vi "MDriveCommand.vi"(4 "Channel Name":string, 6 "Port Name":string, 8 "Numeric Value":dbl format="%.2f", 9 "MDriveCommand":T2="DePowerMotor", 10 "Address":i8) -> (0 "String Reply":string, 1 "Error Description":string, 2 "Numeric Reply":dbl, 3 "OK":bool)   [LabVIEW 2020]
uses:
  MDriveDriveCommand.ctl
  CommandDescriptor.ctl
  ~subVIs/CommandPhases.ctl
  ~subVIs/GenericDriveCommand.ctl
panel:
  out "CommandDescriptorOutput":T1
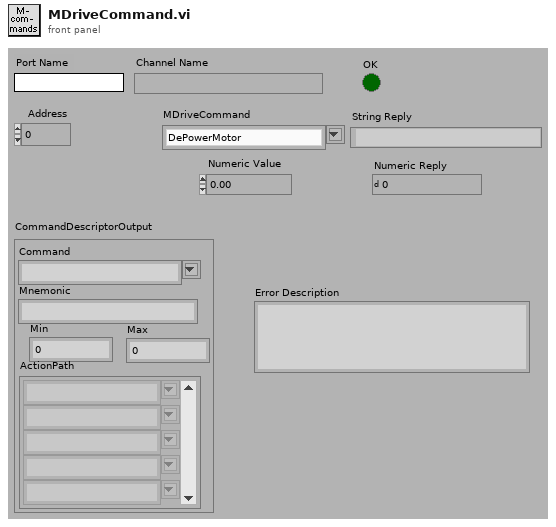
[diagram p1: front panel]
types:
  T1 = typedef "CommandDescriptor.ctl" = cluster{"Command":T2, "Mnemonic":string, "Min":dbl, "Max":dbl, "ActionPath":T3[]}
  T2 = typedef "MDriveDriveCommand.ctl" = string
  T3 = typedef "CommandPhases.ctl" = string
  T4 = typedef "GenericDriveCommand.ctl" = string
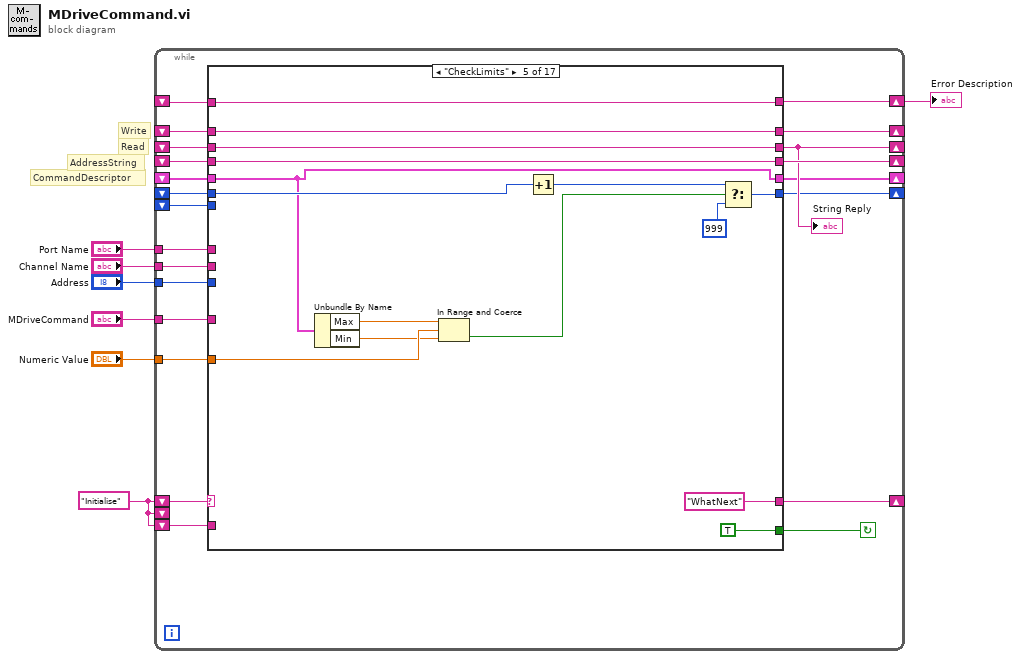
[diagram p0: block diagram]
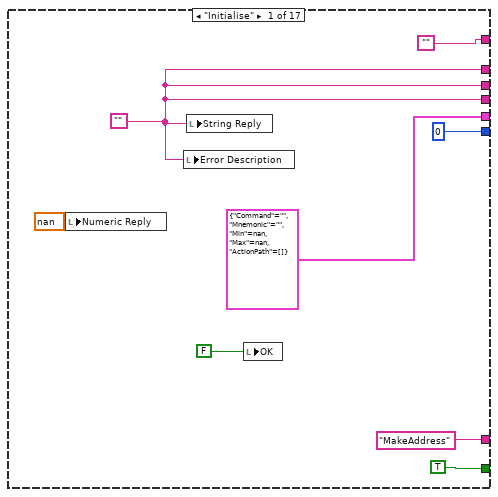
[diagram p2: hidden frame]
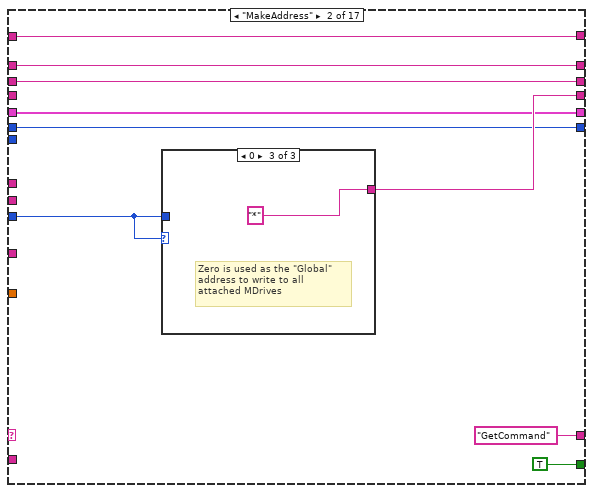
[diagram p3: hidden frame]
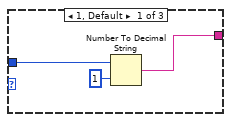
[diagram p4: hidden frame]
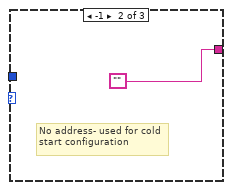
[diagram p5: hidden frame]
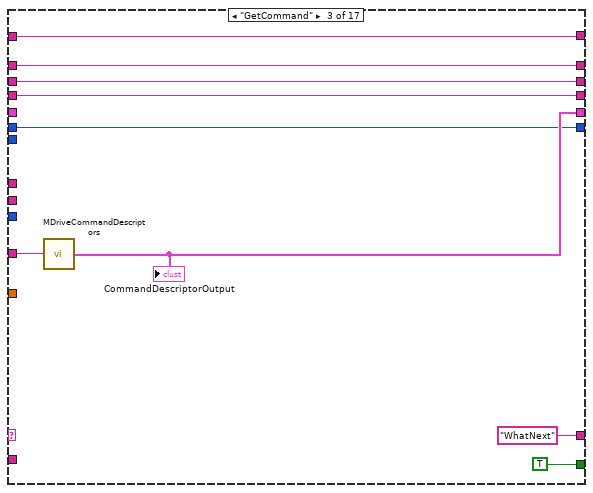
[diagram p6: hidden frame]
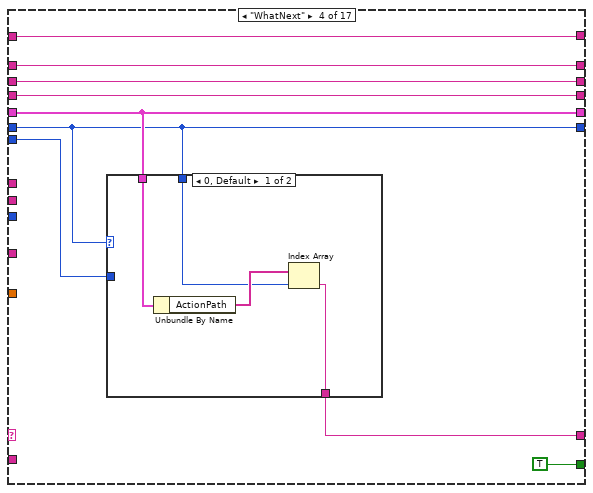
[diagram p7: hidden frame]
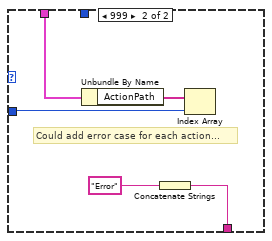
[diagram p8: hidden frame]
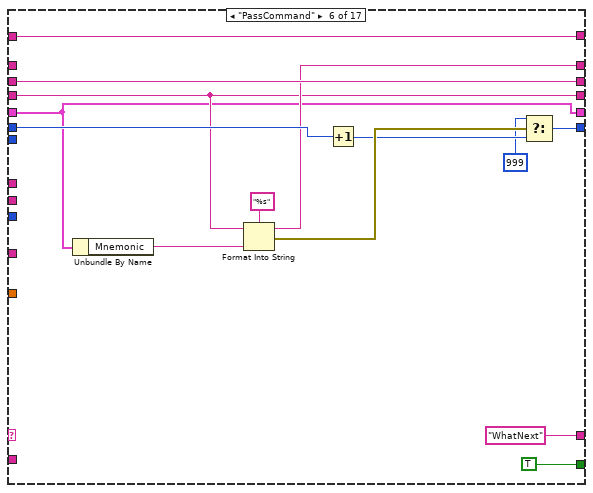
[diagram p9: hidden frame]
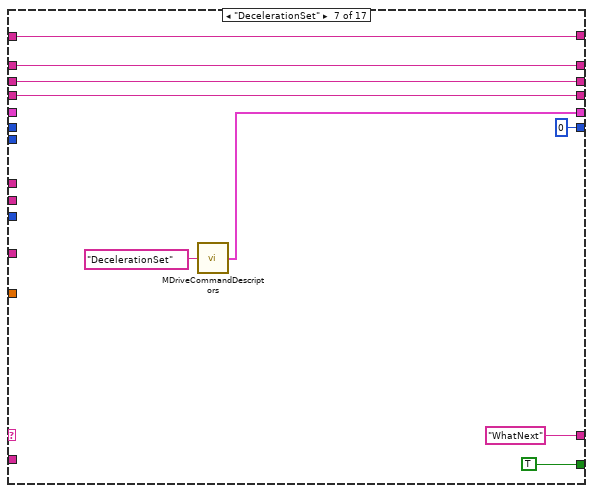
[diagram p10: hidden frame]
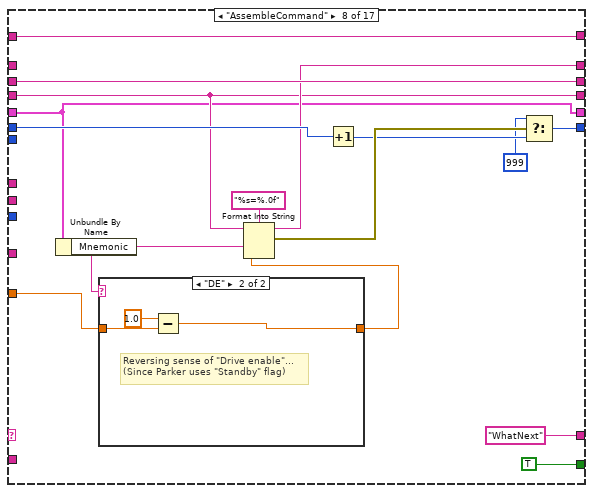
[diagram p11: hidden frame]
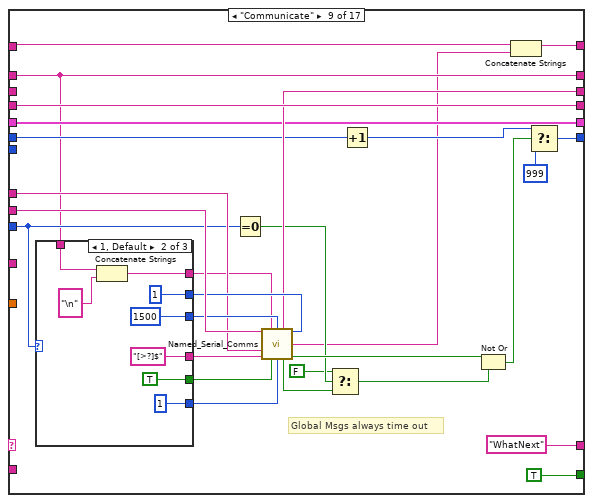
[diagram p13: hidden frame]
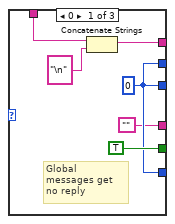
[diagram p14: hidden frame]
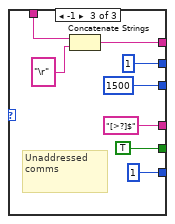
[diagram p15: hidden frame]
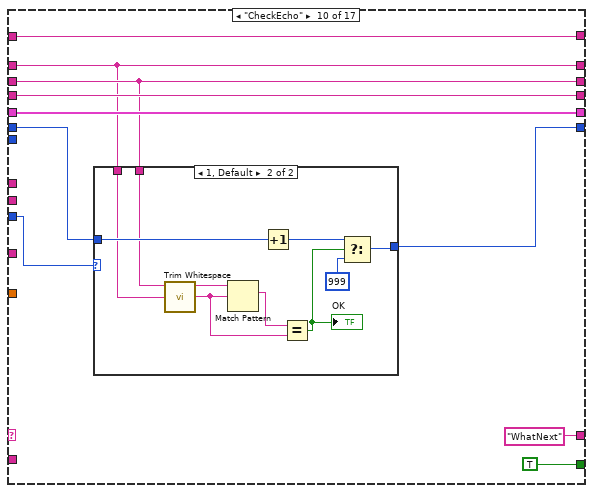
[diagram p16: hidden frame]
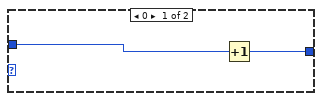
[diagram p17: hidden frame]
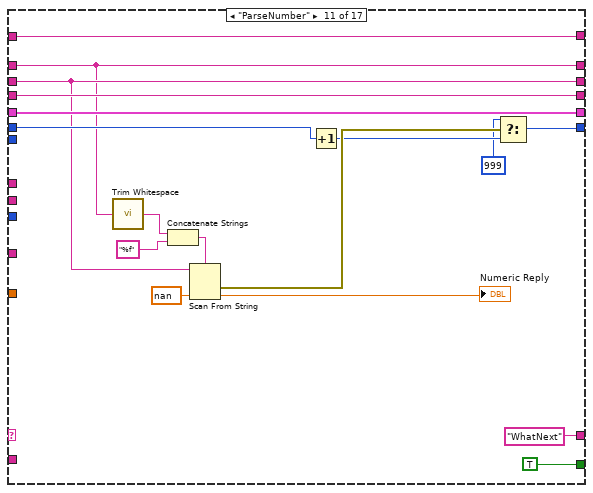
[diagram p18: hidden frame]
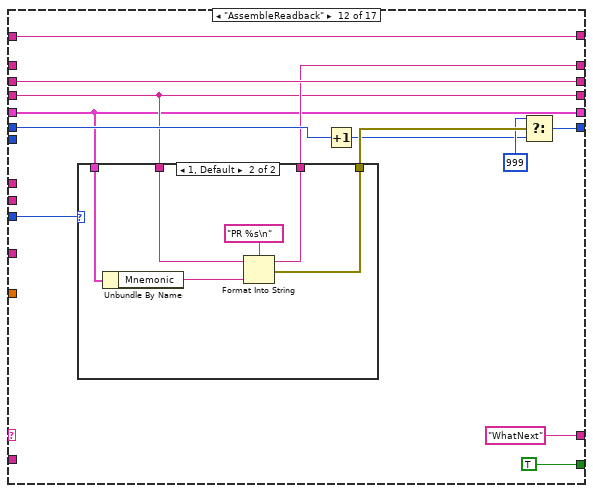
[diagram p19: hidden frame]
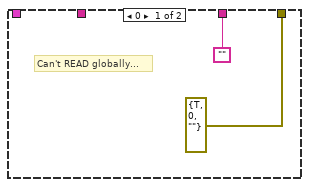
[diagram p20: hidden frame]
diagram:
  w2 = "Initialise"
  # "CommandDescriptor"
  # "AddressString"
  # "Read"
  # "Write"
  n1 = while {
    shift-right: [w18] -> _
    shift-left: w2 -> [w12]
    tunnel: "Address" -> [w29]
    tunnel: "MDriveCommand" -> [w28]
    tunnel: "Numeric Value" -> [w27]
    shift-right: [w26] -> _
    shift-left: _ -> [w25]
    tunnel: "Port Name" -> [w24]
    tunnel: "Channel Name" -> [w23]
    shift-right: [w17] -> _
    shift-left: _ -> [w22]
    shift-right: [w20] -> _
    shift-left: _ -> [w19]
    shift-right: [w16] -> _
    shift-left: _ -> [w15]
    shift-right: [w13] -> _
    shift-left: _ -> [w14]
    shift-left: _ -> [w11]
    shift-left: w2 -> [_]
    shift-left: w2 -> [w10]
    shift-right: [w8] -> w1
    shift-left: _ -> [w9]
    stop <- w21 continue-if-true
    n2 = case shown="\"CheckLimits\"" w12 {
      selector: w12 -> [_ _ _ _ _ _ _ _ _ _ _ _ _ _ _ _ w324]
      tunnel: ["MakeAddress" "GetCommand" "WhatNext" w65 "WhatNext" "WhatNext" "WhatNext" "WhatNext" "WhatNext" "WhatNext" "WhatNext" "WhatNext" w250 "Error" "Initialise" "Initialise" w324] -> w18
      tunnel: w29 -> [_ w39 _ _ _ _ _ _ w142 w188 _ w229 _ _ _ _ _]
      tunnel: w28 -> [_ _ w57 _ _ _ _ _ _ _ _ _ _ _ _ _ _]
      tunnel: w27 -> [_ _ _ _ w91 _ _ w119 _ _ _ _ _ _ _ w311 _]
      tunnel: [w32 w44 w59 w68 w89 w102 w110 w127 w141 w189 w211 w232 w256 w274 w303 w316 w322] -> w26
      tunnel: w25 -> [_ w44 w59 w68 w89 _ w110 _ w141 w189 w211 _ w256 w274 w296 _ _]
      tunnel: w24 -> [_ _ _ _ _ _ _ _ w158 _ _ _ _ _ w297 _ _]
      tunnel: w23 -> [_ _ _ _ _ _ _ _ w164 _ _ _ _ w269 w298 _ _]
      tunnel: [w32 w43 w58 w67 w93 w107 w116 w132 w155 w190 w218 w237 w254 w279 w303 w316 w322] -> w17
      tunnel: w22 -> [_ w43 w58 w67 w93 w107 w116 w132 _ w190 w218 w237 w254 w279 w295 _ _]
      tunnel: [TRUE TRUE ("Continue") TRUE ("Continue") TRUE ("Continue") TRUE TRUE TRUE TRUE TRUE TRUE TRUE TRUE w251 TRUE FALSE ("Continue") FALSE ("Continue") FALSE] -> w21
      tunnel: [w32 w46 w56 w66 w92 w101 w113 w126 w156 w195 w223 w230 w255 w284 w303 w316 w322] -> w20
      tunnel: w19 -> [_ _ w56 w66 w92 w101 w113 w126 w156 w195 w223 w230 w255 w284 _ w309 _]
      tunnel: [T1 {"Command"="", "Mnemonic"="", "Min"=nan, "Max"=nan, "ActionPath"=[]} ("CommandDescriptorOutput") w41 w54 w64 w80 w98 w112 w124 w154 w191 w219 w228 w248 w280 w302 w314 w321] -> w16
      tunnel: w15 -> [_ w41 _ w64 w80 w98 _ w124 w154 w191 w219 w228 w247 w280 w302 w314 w321]
      tunnel: w14 -> [_ w40 w53 w63 w84 w103 _ w128 w149 w192 w220 w233 _ w281 w301 w315 w320]
      tunnel: [0 w40 w53 w63 w85 w104 0 ("f") w129 w151 w193 w221 w234 0 ("f") w282 w301 w315 w320] -> w13
      tunnel: w11 -> [_ _ _ w62 _ _ _ _ _ _ _ _ _ _ _ _ _]
      tunnel: w10 -> [_ _ _ _ _ _ _ _ _ _ _ _ _ _ w293 _ _]
      tunnel: w9 -> [_ w38 w52 w61 w79 w94 w108 w117 w139 w187 w208 w225 w246 w266 w286 w308 w319]
      tunnel: ["" w38 w52 w61 w79 w94 w108 w117 w138 w187 w208 w225 w246 w264 w286 w306 w319] -> w8
      frame "Initialise" {
        w32 = ""
        n3 = local write "Numeric Reply"(nan ("Numeric Reply")) -> ()
        n4 = local write "Error Description"(w32) -> ()
        n5 = local write "String Reply"(w32) -> ()
        n6 = local write "OK"(FALSE ("GoodEcho")) -> ()
      }
      frame "MakeAddress" {
        n7 = case shown="0" w39 {
          tunnel: w39 -> [w48 _ _]
          tunnel: [w47 "" "*"] -> w46
          frame 1, Default {
            n8 = Number To Decimal String(number=w48, width (-)=i16 1) -> (decimal integer string=w47:string)
          }
          frame -1 {
            # "No address- used for cold start configuration"
          }
          frame 0 {
            # "Zero is used as the \"Global\" address to write to all attached MDrives"
          }
        }
      }
      frame "GetCommand" {
        n9 = call "MDriveCommandDescriptors.vi"("MDriveCommand"=w57) -> ("CommandDescriptorOutput"=w54:T1)  [unwired: 4 out]
        "CommandDescriptorOutput" <- w54
      }
      frame "WhatNext" {
        n10 = case shown="0, Default" w63 {
          tunnel: [w72 w75] -> w65
          tunnel: w64 -> [w71 w76]
          tunnel: w63 -> [w70 _]
          tunnel: w62 -> [_ w77]
          frame 0, Default {
            n11 = Unbundle By Name(w71) -> ("ActionPath"=w73:T3[])
            n12 = Index Array(array=w73, index=w70) -> (element=w72:T3)
          }
          frame 999 {
            # "Could add error case for each action..."
            n13 = Unbundle By Name(w76) -> ("ActionPath"=w78:T3[])
            n14 = Concatenate Strings("Error") -> (w75:string)
            n15 = Index Array(array=w78, index=w77) -> ()  [unwired: 1 out]
          }
        }
      }
      frame "CheckLimits" {
        n16 = Unbundle By Name(w80) -> ("Max"=w88:dbl, "Min"=w87:dbl)
        n17 = In Range and Coerce(upper limit=w88, x=w91, lower limit=w87) -> (In Range?=w82:bool)  [unwired: 1 out]
        n18 = Increment(x=w84) -> (x+1=w83:i32)
        n19 = Select(t=w83, s=w82, f=999) -> (s? t:f=w85:i32)
      }
      frame "PassCommand" {
        n20 = Unbundle By Name(w98) -> ("Mnemonic"=w100:string)
        n21 = Format Into String(format string="%s", initial string=w101, w100) -> (resulting string=w102:string, error out=w97:errorcluster)  [unwired: 1 in]
        n22 = Increment(x=w103) -> (x+1=w96:i32)
        n23 = Select(t=999 ("f"), s=w97, f=w96) -> (s? t:f=w104:i32)
      }
      frame "DecelerationSet" {
        n24 = call "MDriveCommandDescriptors.vi"("MDriveCommand"=T4 "DecelerationSet" ("GenericDriveCommand")) -> ("CommandDescriptorOutput"=w112:T1)  [unwired: 4 out]
      }
      frame "AssembleCommand" {
        n25 = Unbundle By Name(w124) -> ("Mnemonic"=w120:string)
        n26 = case shown="\"DE\"" w120 {
          tunnel: w119 -> [w133 w136]
          tunnel: [w133 w134] -> w118
          frame "False", Default {
          }
          frame "DE" {
            # "Reversing sense of \"Drive enable\"...\n(Since Parker uses \"Standby\" flag)"
            n27 = Subtract(x=1.0, y=w136) -> (x-y=w134:dbl)
          }
        }
        n28 = Format Into String(format string="%s=%.0f", initial string=w126, w120, w118) -> (resulting string=w127:string, error out=w123:errorcluster)  [unwired: 1 in]
        n29 = Increment(x=w128) -> (x+1=w122:i32)
        n30 = Select(t=999 ("f"), s=w123, f=w122) -> (s? t:f=w129:i32)
      }
      frame "Communicate" {
        # "Global Msgs always time out"
        n31 = case shown="1, Default" w142 {
          tunnel: ["" "[>?]$" "[>?]$"] -> w163
          tunnel: [w169 1 ("Terminate Count") 1 ("Terminate Count")] -> w162
          tunnel: [w169 u32 1500 ("Timeout/ms") u32 1500 ("Timeout/ms")] -> w161
          tunnel: [TRUE ("Log Errors?") TRUE ("Log Errors?") TRUE ("Log Errors?")] -> w160
          tunnel: [w169 1 ("!Error retries") 1 ("!Error retries")] -> w159
          tunnel: w141 -> [w165 w173 w181]
          tunnel: [w166 w172 w180] -> w140
          frame 0 {
            w169 = 0 ("!Error retries")
            # "Global messages get no reply"
            n32 = Concatenate Strings(w165, "\n" ("string")) -> (w166:string)
          }
          frame 1, Default {
            n33 = Concatenate Strings(w173, "\n" ("string")) -> (w172:string)
          }
          frame -1 {
            # "Unaddressed comms"
            n34 = Concatenate Strings(w181, "\r" ("string")) -> (w180:string)
          }
        }
        n35 = Equal To 0?(x=w142) -> (x = 0?=w145:bool)
        n36 = call "Named_Serial_Comms.vi"("Channel Name"=w164, "Write"=w140, "Timeout/ms"=w161, "!Error retries"=w159, "Port Name"=w158, "Term Grep"=w163, "Log Errors?"=w160, "Terminate Count"=w162) -> ("Read"=w155:string, "Error Description"=w137:string, "Timed out"=w144:bool, "Serial Error"=w152:bool)  [unwired: 1 in, 3 out]
        n37 = Select(t=FALSE, s=w145, f=w144) -> (s? t:f=w146:bool)
        n38 = Increment(x=w149) -> (x+1=w148:i32)
        n39 = Not Or(1:w146, 2:w152) -> (0:w150:bool)
        n40 = Concatenate Strings(w139, w137) -> (w138:string)
        n41 = Select(t=w148, s=w150, f=999) -> (s? t:f=w151:i32)
      }
      frame "CheckEcho" {
        n42 = case shown="1, Default" w188 {
          tunnel: [w197 w206] -> w193
          tunnel: w192 -> [w198 w203]
          tunnel: w190 -> [_ w201]
          tunnel: w189 -> [_ w200]
          frame 0 {
            n43 = Increment(x=w198) -> (x+1=w197:i32)
          }
          frame 1, Default {
            n44 = call <vilib>:"Trim Whitespace.vi"("string"=w200) -> ("trimmed string"=w199:string)  [unwired: 1 in]
            n45 = Match Pattern(string=w201, regular expression=w199) -> (match substring=w202:string)  [unwired: 4 out]
            n46 = Increment(x=w203) -> (x+1=w204:i32)
            n47 = Equal?(x=w202, y=w199) -> (x = y?=w205:bool)
            "OK" <- w205
            n48 = Select(t=w204, s=w205, f=999) -> (s? t:f=w206:i32)
          }
        }
      }
      frame "ParseNumber" {
        n49 = call <vilib>:"Trim Whitespace.vi"("string"=w211) -> ("trimmed string"=w209:string)  [unwired: 1 in]
        n50 = Concatenate Strings(w209, "%f" ("format string")) -> (w212:string)
        n51 = Scan From String(format string=w212, input string=w218, default 1=nan ("default value 1")) -> (error out=w216:errorcluster, output 1=→"Numeric Reply":dbl)  [unwired: 2 in, 2 out]
        n52 = Increment(x=w220) -> (x+1=w215:i32)
        n53 = Select(t=999, s=w216, f=w215) -> (s? t:f=w221:i32)
      }
      frame "AssembleReadback" {
        n54 = case shown="1, Default" w229 {
          tunnel: w228 -> [_ w245]
          tunnel: ["" w244] -> w232
          tunnel: [errorcluster {"status"=TRUE, "code"=0, "source"=""} ("error IO") w243] -> w231
          tunnel: w230 -> [_ w242]
          frame 0 {
            # "Can't READ globally..."
          }
          frame 1, Default {
            n55 = Unbundle By Name(w245) -> ("Mnemonic"=w241:string)
            n56 = Format Into String(format string="PR %s\n", initial string=w242, w241) -> (resulting string=w244:string, error out=w243:errorcluster)  [unwired: 1 in]
          }
        }
        n57 = Increment(x=w233) -> (x+1=w226:i32)
        n58 = Select(t=999 ("f"), s=w231, f=w226) -> (s? t:f=w234:i32)
      }
      frame "Done" {
        n59 = Match Pattern(string=w254, regular expression="?") -> (offset past match=w249:i32)  [unwired: 4 out]
        n60 = case shown="-1" w249 {
          tunnel: [TRUE ("Continue") FALSE ("Continue")] -> w251
          tunnel: ["WhatNext" "Initialise"] -> w250
          tunnel: [w259 w261] -> w248
          tunnel: w247 -> [_ w261]
          frame 0, Default {
            n61 = call "MDriveCommandDescriptors.vi"("MDriveCommand"=T4 "GetError" ("GenericDriveCommand")) -> ("CommandDescriptorOutput"=w259:T1)  [unwired: 4 out]
          }
          frame -1 {
          }
        }
      }
      frame "ParseError" {
        n62 = call <vilib>:"Trim Whitespace.vi"("string"=w274) -> ("trimmed string"=w272:string)  [unwired: 1 in]
        n63 = Concatenate Strings(w272, "%s" ("format string")) -> (w275:string)
        n64 = Scan From String(format string=w275, input string=w279, default 1="") -> (error out=w278:errorcluster, output 1=w270:string)  [unwired: 2 in, 2 out]
        n65 = call "MDriveErrorCodes.vi"("Error Code"=w270) -> ("Error Description"=w268:string)  [unwired: 4 out]
        n66 = Increment(x=w281) -> (x+1=w277:i32)
        n67 = Format Into String(format string="The %s has %s", w269, w268) -> (resulting string=w265:string)  [unwired: 2 in, 1 out]
        n68 = Concatenate Strings(w266, w265) -> (w264:string)
        n69 = Select(t=999, s=w278, f=w277) -> (s? t:f=w282:i32)
      }
      frame "Error" {
        w290 = "Error in MDriveCommand.vi: " ("string")
        w303 = ""
        n70 = local read "Error Description"() -> (w289:string)
        n71 = call "Serial_log_build.vi"("Read"=w295, "Write String"=w296, "Port Name"=w297) -> ("Output Array"=w299:string[])
        n72 = Empty String/Path?(string/path=w289) -> (empty?=w294:bool)
        n73 = Concatenate Strings(w290, w293) -> (w292:string)
        n74 = Concatenate Strings(w290, w289) -> (w291:string)
        n75 = Select(t=w292, s=w294, f=w291) -> (s? t:f=w288:string)
        n76 = call "Write_serial_log.vi"("Log Type"="MDrive_Error_Log", "Log Array"=w299, "Header message"=w288, "Channel Name"=w298) -> ()  [unwired: 1 out]
        n77 = local write "OK"(FALSE ("GoodEcho")) -> ()
      }
      frame "CheckLimitsError" {
        w316 = ""
        n78 = Unbundle By Name(w314) -> ("Mnemonic"=w312:string)
        n79 = Format Into String(format string="%s=%.0f) to drive %s", initial string="Attempt to Write an out-of-range value (" ("message"), w312, w311, w309) -> (resulting string=w307:string)  [unwired: 1 in, 1 out]
        n80 = Concatenate Strings(w308, w307) -> (w306:string)
      }
      frame "NoMatch", Default {
        w322 = ""
        n81 = One Button Dialog(message="Case not found in MDriveCommands.vi", button name ("OK")="Oh Bugger...") -> ()  [unwired: 1 out]
      }
    }
    "String Reply" <- w17
  }
  "Error Description" <- w1
